vi "OB Write.vi"(7 "WriteDataLen":u32, 9 "pWriteData":T1, 10 "Channel":u8, 11 "DevHandle":i32) -> (1 "pWriteData out":T1, 3 "function return":i32)   [LabVIEW 2010, in "usb2openbus.lvlib"]
doc: "int WINAPI OB_Write(int DevHandle, unsigned char Channel,OB_DATA *pWriteData,unsigned int WriteDataLen);"
uses:
  usb2openbus.lvlib
  USB2XXX.dll
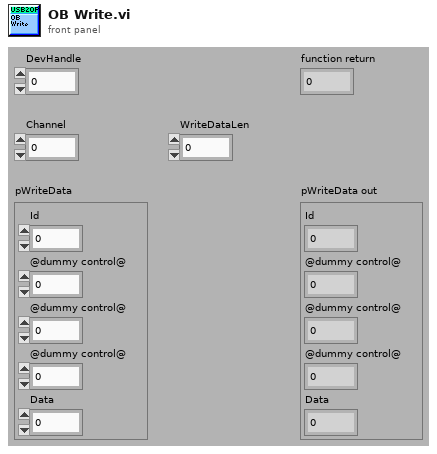
[diagram p1: front panel]
types:
  T1 = cluster{"Id":i8, "@dummy control@":i8, "@dummy control@":i8, "@dummy control@":i8, "Data":u32}
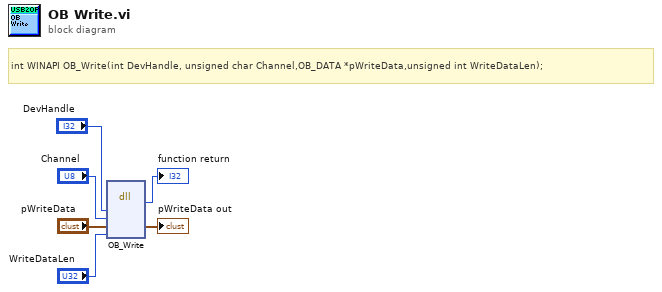
[diagram p0: block diagram]
diagram:
  # "int WINAPI OB_Write(int DevHandle, unsigned char Channel,OB_DATA *pWriteData,unsigned int WriteDataLen);"
  n1 = dll-call lib="F:/OtherWork/STM32/USB2XXX_Example/trunk/Labview/PublicFiles/usb2openbus/USB2XXX.*" fn="OB_Write"("DevHandle"="DevHandle", "Channel"="Channel", "pWriteData"="pWriteData", "WriteDataLen"="WriteDataLen") -> (→"function return":i32, "pWriteData"=→"pWriteData out":T1)  [unwired: 6 in, 2 out]
